vi "cm2nm_start_new_session_info.vi"(1 "Session Name/ID_out":string, 2 "Sample_Information":T1, 3 "Instrument_out":u16, 4 "Session File_out":path) -> (0 "Sample_out":T1)   [LabVIEW 2011]
doc: "Initialize the sample out variable with the new current session information."
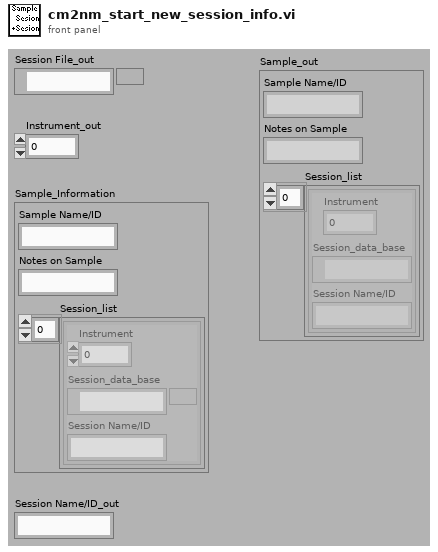
[diagram p1: front panel]
types:
  T1 = cluster{"Sample Name/ID":string, "Notes on Sample":string, "Session_list":cluster{"Instrument":u16, "Session_data_base":path, "Session Name/ID":string}[]}
  T2 = cluster{"Instrument":u16, "Session_data_base":path, "Session Name/ID":string}
  T3 = cluster{"Instrument":u16, "Session_data_base":path, "Session Name/ID":string}[]
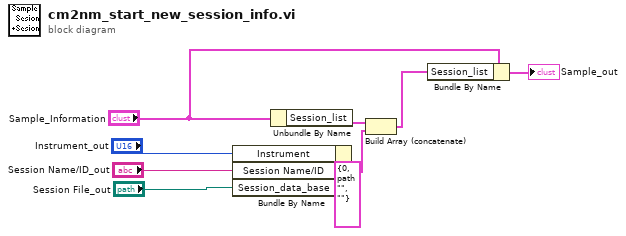
[diagram p0: block diagram]
diagram:
  n1 = Bundle By Name(cluster=T2 {"Instrument"=0, "Session_data_base"=path "", "Session Name/ID"=""} ("input cluster"), "Instrument"="Instrument_out", "Session Name/ID"="Session Name/ID_out", "Session_data_base"="Session File_out") -> (w4:T2)
  n2 = Unbundle By Name("Sample_Information") -> ("Session_list"=w2:T3)
  n3 = Build Array (concatenate)(w2, w4) -> (w5:T3)
  n4 = Bundle By Name(cluster="Sample_Information", "Session_list"=w5) -> (→"Sample_out":T1)
